vi "increment2.vi"(4 "State":i16, 5 "Time":dbl format="%.2f", 6 "Sensor Values":dbl[](array[numeric]), 7 "Set Points":dbl[](array[numeric])) -> (0 "required data":T1={"Set Point names"=["reset state", "state to increment", "slope", "intercept", "max x"], "required number of setpoints"=5, "required number of sensors"=0, "Sensor names"=[]}, 3 "output value":dbl)   [LabVIEW 2019]
panel:
  # "Enter the correct information for this control code in the required data structure below. Then make the current value default by right clicking on the border of the data structure. Select \"data operations\" and then select \"make current value default\". These values will be displayed by process controller."
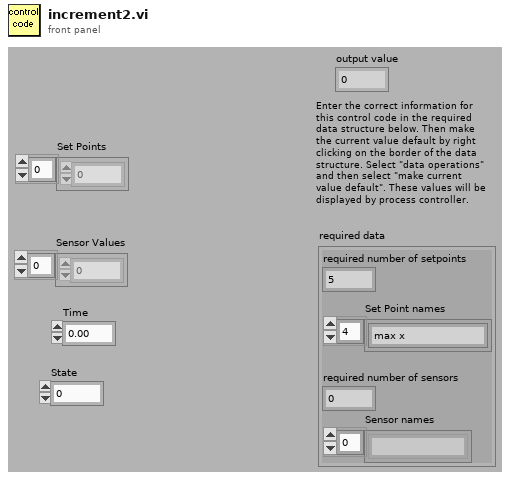
[diagram p1: front panel]
types:
  T1 = cluster{"Set Point names":string[], "required number of setpoints":u8, "required number of sensors":u8, "Sensor names":string[]}
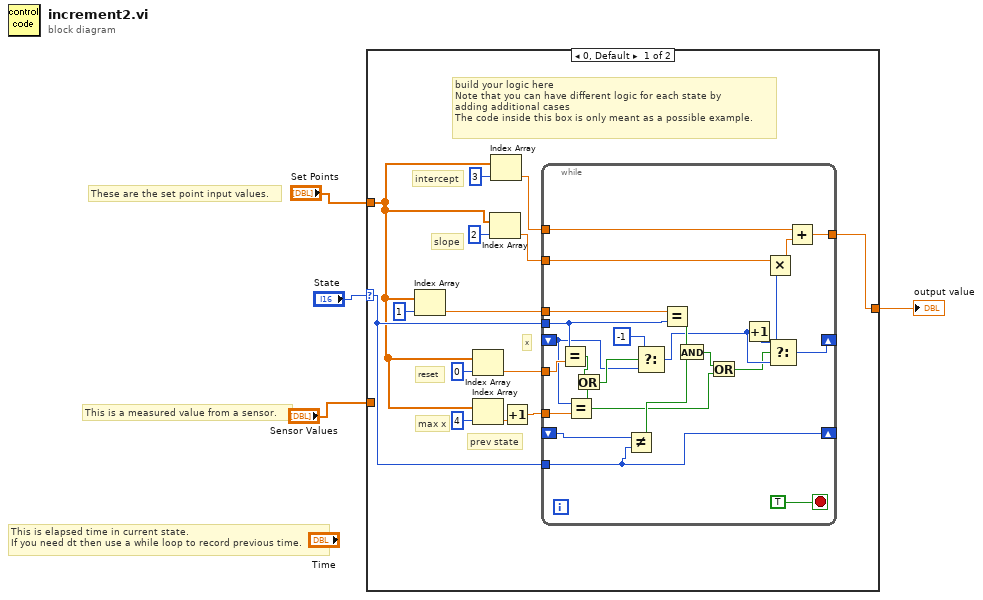
[diagram p0: block diagram]
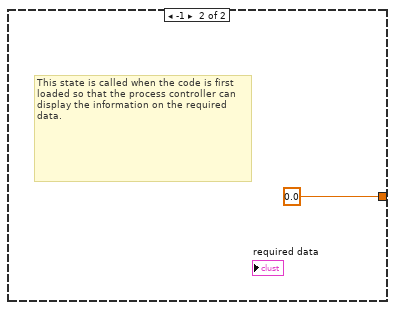
[diagram p2: hidden frame]
diagram:
  # "These are the set point input values."
  # "This is a measured value from a sensor."
  # "This is elapsed time in current state.\nIf you need dt then use a while loop to record previous time."
  n1 = case shown="0, Default" "State" {
    selector: "State" -> [w15 _]
    tunnel: [w11 0.0 ("fraction on")] -> w3
    tunnel: "Set Points" -> [w7 _]
    tunnel: "Sensor Values" -> [_ _]
    frame 0, Default {
      # "max x"
      # "prev state"
      # "reset"
      # "intercept"
      # "slope"
      # "x"
      # "build your logic here\nNote that you can have different logic for each state by\nadding additional cases\nThe code inside this box is only meant as a possible example."
      n2 = Index Array(array=w7, index=1) -> (element=w16:dbl)
      n3 = Index Array(array=w7, index=0) -> (element=w9:dbl)
      n4 = Index Array(array=w7, index=4) -> (element=w6:dbl)
      n5 = Index Array(array=w7, index=2) -> (element=w13:dbl)
      n6 = Index Array(array=w7, index=3) -> (element=w12:dbl)
      n7 = Increment(x=w6) -> (x+1=w5:dbl)
      n8 = while {
        shift-right: [w40] -> _
        shift-left: _ -> [w27]
        tunnel: w15 -> [w40]
        tunnel: w16 -> [w41]
        tunnel: w15 -> [w30]
        shift-right: [w38] -> _
        shift-left: _ -> [w23]
        tunnel: w13 -> [w34]
        tunnel: w12 -> [w37]
        tunnel: [w36] -> w11
        tunnel: w9 -> [w29]
        tunnel: w5 -> [w26]
        stop <- TRUE stop-if-true
        n9 = Equal?(x=w30, y=w29) -> (x = y?=w25:bool)
        n10 = Equal?(x=w23, y=w26) -> (x = y?=w20:bool)
        n11 = Or(x=w25, y=w20) -> (x .or. y?=w24:bool)
        n12 = Not Equal?(x=w27, y=w40) -> (x != y?=w39:bool)
        n13 = Select(t=-1, s=w24, f=w23) -> (s? t:f=w28:i32)
        n14 = Equal?(x=w41, y=w30) -> (x = y?=w33:bool)
        n15 = And(x=w33, y=w39) -> (x .and. y?=w21:bool)
        n16 = Or(x=w21, y=w20) -> (x .or. y?=w19:bool)
        n17 = Increment(x=w28) -> (x+1=w32:i32)
        n18 = Select(t=w32, s=w19, f=w28) -> (s? t:f=w38:i32)
        n19 = Multiply(x=w34, y=w38) -> (x*y=w31:dbl)
        n20 = Add(x=w37, y=w31) -> (x+y=w36:dbl)
      }
    }
    frame -1 {
      # "This state is called when the code is first loaded so that the process controller can display the information on the required data."
    }
  }
  "output value" <- w3
